vi "Spawn Root.vi"(6 "UID":string, 9 "Persistent Layers":refnum<class "Actor.lvclass">[](array[class]), 10 "Local Layers":refnum<class "Actor.lvclass">[](array[class])) -> (0 "Error out":errorcluster, 5 "Actor out":refnum<class "Actor.lvclass">)   [LabVIEW 2025, in "jettl.lvlib"]
uses:
  jettl.lvlib
  Actor/Actor.lvclass
  Error/Error.lvlib
  Core Actor/Core Actor.lvlib
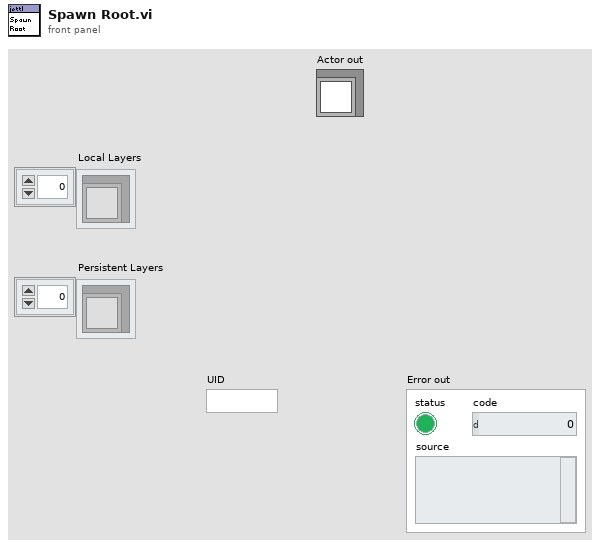
[diagram p1: front panel]
types:
  T1 = typedef "jettl.lvlib/Child UIDs.ctl" = set{string}
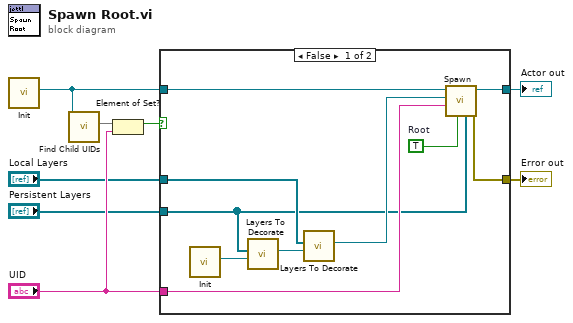
[diagram p0: block diagram]
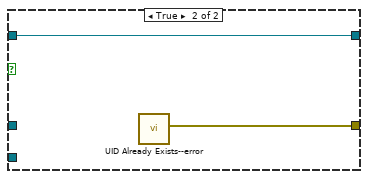
[diagram p2: hidden frame]
diagram:
  n1 = call "Init.vi"() -> ("Actor"=w1:refnum<class "Actor.lvclass">)  [unwired: 11 in]
  n2 = call-dynamic "Find Child UIDs.vi"("Actor in"=w1) -> ("Child UIDs"=w8:T1)  [unwired: 10 in]
  n3 = Element of Set?(10:"UID", 11:w8) -> (3:w7:bool)
  n4 = case shown="False" w7 {
    tunnel: w1 -> [w15 w20]
    tunnel: [w16 w19] -> w6
    tunnel: [w17 w20] -> w5
    tunnel: "UID" -> [w14 _]
    tunnel: "Local Layers" -> [w13 _]
    tunnel: "Persistent Layers" -> [w9 _]
    frame False {
      w10 = TRUE  # Root
      n5 = call "Init.vi"() -> ("Actor"=w18:refnum<class "Actor.lvclass">)  [unwired: 11 in]
      n6 = call "Layers To Decorate.vi"("Actor To Decorate"=w18, "Layers"=w9) -> ("Decorated Actor"=w12:refnum<class "Actor.lvclass">)  [unwired: 9 in]
      n7 = call "Layers To Decorate.vi"("Actor To Decorate"=w12, "Layers"=w13) -> ("Decorated Actor"=w11:refnum<class "Actor.lvclass">)  [unwired: 9 in]
      n8 = call-dynamic "Spawn.vi"("Persistent Layers"=w9, "Root"=w10, "UID"=w14, "Unified Actor"=w11, "Actor in"=w15) -> ("Error out"=w16:errorcluster, "Actor out"=w17:refnum<class "Actor.lvclass">)  [unwired: 5 in]
    }
    frame True {
      n9 = call "UID Already Exists--error.vi"() -> ("Error"=w19:errorcluster)  [unwired: 11 in]
    }
  }
  "Error out" <- w6
  "Actor out" <- w5
